vi "Arinst SSA-TG.vi"() -> ()   [LabVIEW 2015]
doc: "Example VI that demonstrates all library features."
uses:
  PL Arinst SSA-TG.lvclass
panel:
  out "scan time, ms":u32
  out "SSA-TG":refnum<class "PL Arinst SSA-TG.lvclass">
  in  "scan":T1={"start, Hz"=1000000000, "end, Hz"=2000000000, "step, Hz"=100000000, "attenuation, dB"=0.0, "scan"=FALSE, "with tracking"=FALSE} {"step, Hz" format="%.0p"; "end, Hz" format="%.0p"; "start, Hz" format="%.0p"}
  in  "power, dBm":dbl=-25.0
  in  "frequency, Hz":u32=1000000000 format="%.0p"
  in  "turn generator off":bool
  in  "turn generator on":bool
  out "scan graph":T2(graph)
  in  "port":refnum<visa-resource-name>
  out "error":errorcluster
  in  "stop":bool
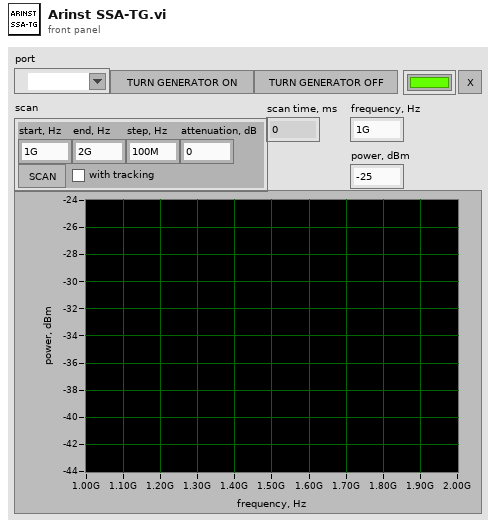
[diagram p1: front panel]
types:
  T1 = cluster{"start, Hz":u32, "end, Hz":u32, "step, Hz":u32, "attenuation, dB":dbl, "scan":bool, "with tracking":bool}
  T2 = cluster{"start, Hz":u32, "step, Hz":u32, "amplitude, dBm":dbl[]}
  T3 = cluster{"start, Hz":u32, "step, Hz":u32, "power, dBm":dbl[]}
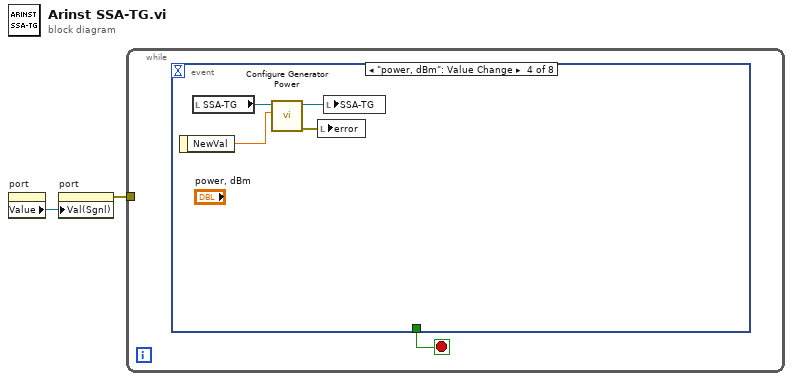
[diagram p0: block diagram]
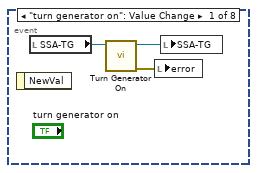
[diagram p2: hidden frame]
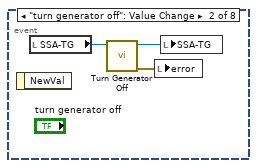
[diagram p3: hidden frame]
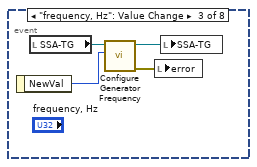
[diagram p4: hidden frame]
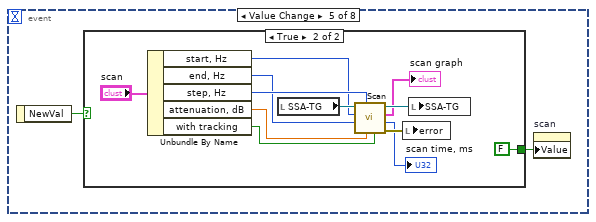
[diagram p5: hidden frame]
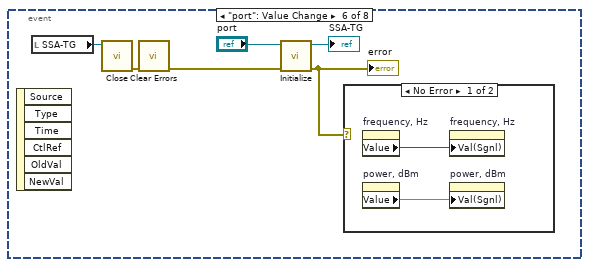
[diagram p7: hidden frame]
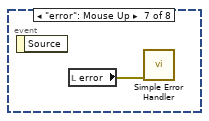
[diagram p9: hidden frame]
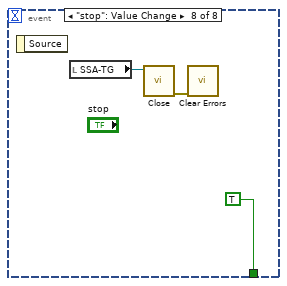
[diagram p10: hidden frame]
diagram:
  n1 = property on="port" class="VISAName"() -> ("Value"=w1:refnum<visa-resource-name>)  [unwired: 2 in, 2 out]
  n2 = property on="port" class="VISAName"("Val(Sgnl)"=w1) -> (error out=w2:errorcluster)  [unwired: 2 in, 1 out]
  n3 = while {
    tunnel: w2 -> [_]
    stop <- w3 stop-if-true
    n4 = event shown="[3] \"power, dBm\": Value Change" {
      selector: _ -> [_ _ _ _ _ _ _ _]
      dyn-events: _ -> [_ _ _ _ _ _ _ _]
      timeout: _ -> [_ _ _ _ _ _ _ _]
      tunnel: [_ _ _ _ _ _ _ TRUE ("stop")] -> w3
      event "turn generator on": Value Change {
        n5 = event-data() -> ()  [unwired: 1 in, 1 out]
        n6 = local read "SSA-TG"() -> (w5:refnum<class "PL Arinst SSA-TG.lvclass">)
        n7 = call "Turn Generator On.vi"("Arinst SSA-TG in"=w5) -> ("error out"=w4:errorcluster, "Arinst SSA-TG out"=w6:refnum<class "PL Arinst SSA-TG.lvclass">)  [unwired: 9 in]
        n8 = local write "error"(w4) -> ()
        n9 = local write "SSA-TG"(w6) -> ()
      }
      event "turn generator off": Value Change {
        n10 = event-data() -> ()  [unwired: 1 in, 1 out]
        n11 = local read "SSA-TG"() -> (w9:refnum<class "PL Arinst SSA-TG.lvclass">)
        n12 = call "Turn Generator Off.vi"("Arinst SSA-TG in"=w9) -> ("error out"=w7:errorcluster, "Arinst SSA-TG out"=w8:refnum<class "PL Arinst SSA-TG.lvclass">)  [unwired: 9 in]
        n13 = local write "error"(w7) -> ()
        n14 = local write "SSA-TG"(w8) -> ()
      }
      event "frequency, Hz": Value Change {
        n15 = event-data() -> ("NewVal"=w10:u32)  [unwired: 1 in]
        n16 = local read "SSA-TG"() -> (w13:refnum<class "PL Arinst SSA-TG.lvclass">)
        n17 = call "Configure Generator Frequency.vi"("frequency, Hz"=w10, "Arinst SSA-TG in"=w13) -> ("error out"=w11:errorcluster, "Arinst SSA-TG out"=w12:refnum<class "PL Arinst SSA-TG.lvclass">)  [unwired: 8 in]
        n18 = local write "error"(w11) -> ()
        n19 = local write "SSA-TG"(w12) -> ()
      }
      event "power, dBm": Value Change {
        n20 = event-data() -> ("NewVal"=w14:dbl)  [unwired: 1 in]
        n21 = local read "SSA-TG"() -> (w17:refnum<class "PL Arinst SSA-TG.lvclass">)
        n22 = call "Configure Generator Power.vi"("power, dBm"=w14, "Arinst SSA-TG in"=w17) -> ("error out"=w15:errorcluster, "Arinst SSA-TG out"=w16:refnum<class "PL Arinst SSA-TG.lvclass">)  [unwired: 8 in]
        n23 = local write "error"(w15) -> ()
        n24 = local write "SSA-TG"(w16) -> ()
      }
      event "scan.scan": Value Change {
        n25 = event-data() -> ("NewVal"=w19:bool)  [unwired: 1 in]
        n26 = case shown="True" w19 {
          tunnel: [_ FALSE ("Value")] -> w18
          frame False {
          }
          frame True {
            n27 = Unbundle By Name("scan") -> ("start, Hz"=w25:u32, "end, Hz"=w24:u32, "step, Hz"=w26:u32, "attenuation, dB"=w23:dbl, "with tracking"=w22:bool)
            n28 = local read "SSA-TG"() -> (w29:refnum<class "PL Arinst SSA-TG.lvclass">)
            n29 = call "Scan.vi"("with tracking (true)"=w22, "attenuation, dB (0)"=w23, "step, Hz"=w26, "end, Hz"=w24, "start, Hz"=w25, "Arinst SSA-TG in"=w29) -> ("error out"=w28:errorcluster, "scan time, ms"=→"scan time, ms":u32, "scan data"=→"scan graph":T3, "Arinst SSA-TG out"=w30:refnum<class "PL Arinst SSA-TG.lvclass">)  [unwired: 2 in]
            n30 = local write "error"(w28) -> ()
            n31 = local write "SSA-TG"(w30) -> ()
          }
        }
        n32 = property on="scan" class="Bool (strict)"("Value"=w18) -> ()  [unwired: 2 in, 2 out]
      }
      event "port": Value Change {
        n33 = event-data() -> ()  [unwired: 1 in, 6 out]
        n34 = local read "SSA-TG"() -> (w37:refnum<class "PL Arinst SSA-TG.lvclass">)
        n35 = call "Close.vi"("Arinst SSA-TG in"=w37) -> ("error out"=w35:errorcluster)  [unwired: 10 in]
        n36 = call <vilib>:"Clear Errors.vi"("error in (no error)"=w35) -> ("error out"=w36:errorcluster)  [unwired: 5 in, 1 out]
        n37 = call "Initialize.vi"("error in (no error)"=w36, "port"="port") -> ("error out"=w32:errorcluster, "Arinst SSA-TG out"=→"SSA-TG":refnum<class "PL Arinst SSA-TG.lvclass">)  [unwired: 8 in]
        "error" <- w32
        n38 = case shown="No Error" w32 {
          frame No Error {
            n39 = property on="frequency, Hz" class="DigNum (strict)"() -> ("Value"=w39:u32)  [unwired: 2 in, 2 out]
            n40 = property on="power, dBm" class="DigNum (strict)"() -> ("Value"=w38:dbl)  [unwired: 2 in, 2 out]
            n41 = property on="frequency, Hz" class="DigNum (strict)"("Val(Sgnl)"=w39) -> ()  [unwired: 2 in, 2 out]
            n42 = property on="power, dBm" class="DigNum (strict)"("Val(Sgnl)"=w38) -> ()  [unwired: 2 in, 2 out]
          }
          frame Error {
          }
        }
      }
      event "error": Mouse Up {
        n43 = event-data() -> ()  [unwired: 1 in, 1 out]
        n44 = local read "error"() -> (w40:errorcluster)
        n45 = call <vilib>:"Simple Error Handler.vi"("error in (no error)"=w40) -> ()  [unwired: 4 in, 5 out]
      }
      event "stop": Value Change {
        n46 = event-data() -> ()  [unwired: 1 in, 1 out]
        n47 = local read "SSA-TG"() -> (w42:refnum<class "PL Arinst SSA-TG.lvclass">)
        n48 = call "Close.vi"("Arinst SSA-TG in"=w42) -> ("error out"=w41:errorcluster)  [unwired: 10 in]
        n49 = call <vilib>:"Clear Errors.vi"("error in (no error)"=w41) -> ()  [unwired: 5 in, 2 out]
      }
    }
  }
